vi "IMAQ_Recreate.vi"(4 "error in":errorcluster, 5 "type":T2 items=["Grayscale (U8)", "Grayscale (I16)", "Grayscale (SGL)", "Complex (CSG)", "RGB (U32)", "HSL (U32)", "RGB (U64)", "Grayscale (U16)"], 6 "name":string, 7 "image in":T1) -> (0 "error out":errorcluster, 3 "image out":T1)   [LabVIEW 2010]
doc: "Checks that the given input IMAQ image and returns it unchanged if it has the name and type as specified. If not, allocates a new image and returns that instead.\n\nEnables display of image from previous VI execution instead of reallocating and wiping the data."
uses:
  <vilib>/vision/Image Controls.llb/IMAQ Image.ctl
  Program Files (x86)/National Instruments/LabVIEW 2010/resource/objmgr/IMAQImage.rc
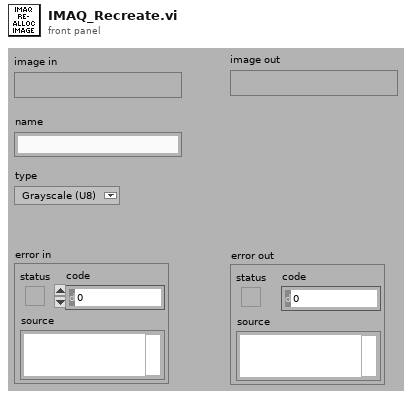
[diagram p1: front panel]
types:
  T1 = typedef "IMAQ Image.ctl" = refnum<image>
  T2 = typedef "Image Type" = u32
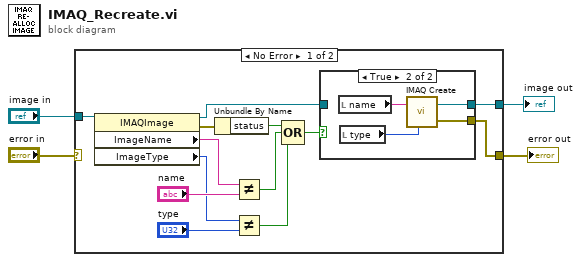
[diagram p0: block diagram]
diagram:
  n1 = case shown="No Error" "error in" {
    selector: "error in" -> [_ w23]
    tunnel: "image in" -> [w17 _]
    tunnel: [w6 _] -> w3
    tunnel: [w5 w23] -> w2
    frame No Error {
      n2 = property class="IMAQImage"(reference=w17) -> (reference out=w7:T1, error out=w16:errorcluster, "ImageName"=w15:string, "ImageType"=w13:i32)  [unwired: 1 in]
      n3 = Unbundle By Name(w16) -> ("status"=w11:bool)
      n4 = Not Equal?(x=w15, y="name") -> (x != y?=w10:bool)
      n5 = Not Equal?(x=w13, y="type") -> (x != y?=w9:bool)
      n6 = Compound Arithmetic op=OR(w11, w10, w9) -> (w8:bool)
      n7 = case shown="True" w8 {
        tunnel: w7 -> [w18 _]
        tunnel: [w18 w20] -> w6
        tunnel: [_ w19] -> w5
        frame False {
        }
        frame True {
          n8 = local read "name"() -> (w22:string)
          n9 = local read "type"() -> (w21:T2)
          n10 = call "IMAQ Create"("Image Name"=w22, "Image Type"=w21) -> ("New Image"=w20:T1, "error out"=w19:errorcluster)  [unwired: 3 in]
        }
      }
    }
    frame Error {
    }
  }
  "image out" <- w3
  "error out" <- w2
